vi "Set index port.vi"(8 "error in (no error)":errorcluster, 9 "Port":cluster{"String":string, "Array 2":bool[]}, 10 "index":i32, 11 "Ports in":refnum<class "Ports.lvclass">) -> (0 "error out":errorcluster, 3 "Ports out":refnum<class "Ports.lvclass">)   [LabVIEW 2019, in "Ports.lvclass"]
uses:
  Ports.lvclass
  Ports.lvclass/Ports.ctl
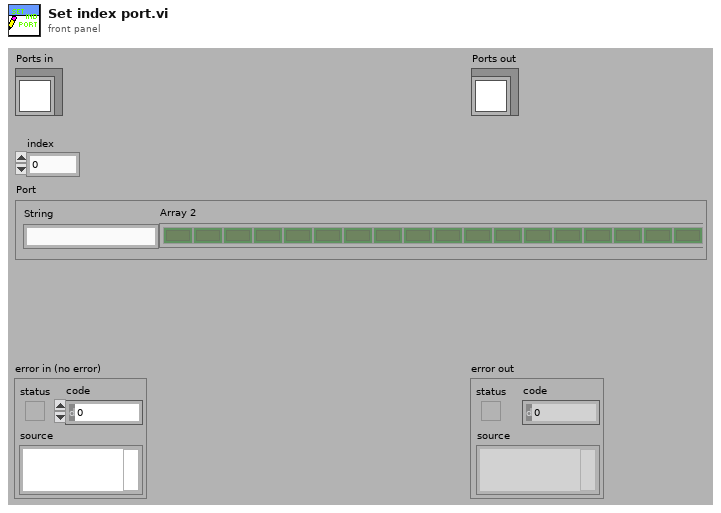
[diagram p1: front panel]
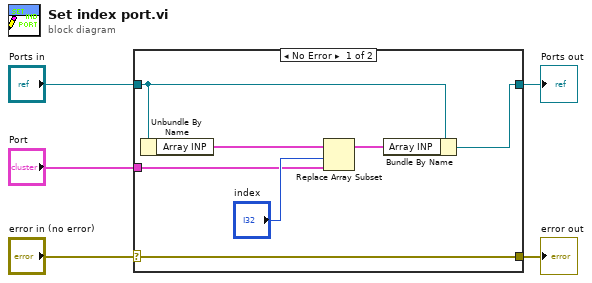
[diagram p0: block diagram]
diagram:
  n1 = case shown="No Error" "error in (no error)" {
    selector: "error in (no error)" -> [w12 w13]
    tunnel: [w12 w13] -> w4
    tunnel: [w11 w14] -> w2
    tunnel: "Ports in" -> [w10 w14]
    tunnel: "Port" -> [w6 _]
    frame No Error {
      n2 = Unbundle By Name(w10) -> ("Array INP"=w9:cluster{"Port Name":string, "Data":bool[]}[])
      n3 = Replace Array Subset(array=w9, new element=w6, index="index") -> (w8:cluster{"Port Name":string, "Data":bool[]}[])
      n4 = Bundle By Name(cluster=w10, "Array INP"=w8) -> (w11:refnum<class "Ports.lvclass">)
    }
    frame Error {
    }
  }
  "error out" <- w4
  "Ports out" <- w2
